vi "Connect To DIAdem.vi"(4 "error in (no error)":errorcluster) -> (0 "error out":errorcluster, 3 "storage refnum":refnum<k20>)   [LabVIEW 2020]
uses:
  <resource>/objmgr/Storage.rc
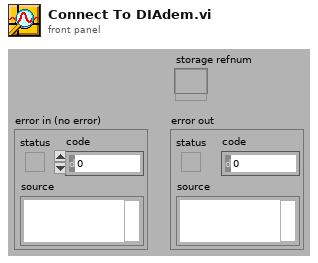
[diagram p1: front panel]
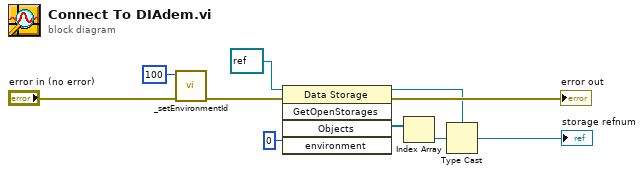
[diagram p0: block diagram]
diagram:
  n1 = call <vilib>:"_setEnvironmentId.vi"("error in (no error)"="error in (no error)", "EnvironmentID"=100) -> ("error out"=w9:errorcluster)  [unwired: 5 out]
  n2 = invoke class="Data Storage" method="GetOpenStorages"(reference=refnum<k20> refnum, error in=w9, "environment"=0) -> (reference out=w6:refnum<k20>, error out=→"error out":errorcluster, "Objects"=w4:refnum<k20>[])  [unwired: 2 in, 2 out]
  n3 = Index Array(array=w4) -> (element=w5:refnum<k20>)  [unwired: 1 in]
  n4 = Type Cast(type=w6, x=w5) -> (*(type *) &x=→"storage refnum":refnum<k20>)
